vi "Draw Compass.vi"(5 "FcdVI Refnum":refnum<vi>, 7 "2D Picture":refnum<vi>, 9 "State in":T1={"Draw Options"={"Outer Border Color"=0, "Inner Border Color"=6316128, "Outer Gradient Color"=2565927, "Inner Gradient Color"=16860, "Compass North Pointer Color"=16711680, "Compass Pointer Color 1"=13355429, "Compass Pointer Color 2"=14934973, "Direction Pointer Color"=16765184, "Text Box Outline Color"=13355429, "Text Box Background Color"=14934973, "Scale Color"=16448250, "Text Color"=0, "Draw Gradient"=TRUE, "Draw Rose"=TRUE, "Simple Scale"=TRUE, "Draw Text"=FALSE, "Font Name"="Helvetica", "Angle Units"=enum."Degrees"}}, 10 "Data in":T4) -> (3 "picture out":picture)   [LabVIEW 2017, in "Compass Indicator.xctl"]
uses:
  <vilib>/robotics/Controls/Compass Indicator/Compass Indicator.xctl
  <vilib>/robotics/Controls/Compass Indicator/_Compass Indicator Support Files/Compass Data.ctl
  <vilib>/robotics/Controls/Compass Indicator/_Compass Indicator Support Files/Compass State.ctl
  <vilib>/robotics/Controls/Compass Indicator/Compass Picture/Draw Options.ctl
  <vilib>/robotics/Controls/Utilities/Angle Units.ctl
  <vilib>/Utility/miscctls.llb/LVBoundsTypeDef.ctl
  <vilib>/Utility/miscctls.llb/LVPositionTypeDef.ctl
  <vilib>/robotics/Controls/Compass Indicator/Compass Picture/NI_Robotics_Compass Picture.lvlib
  <vilib>/robotics/Controls/Utilities/NI_Robotics_Control Utilities.lvlib
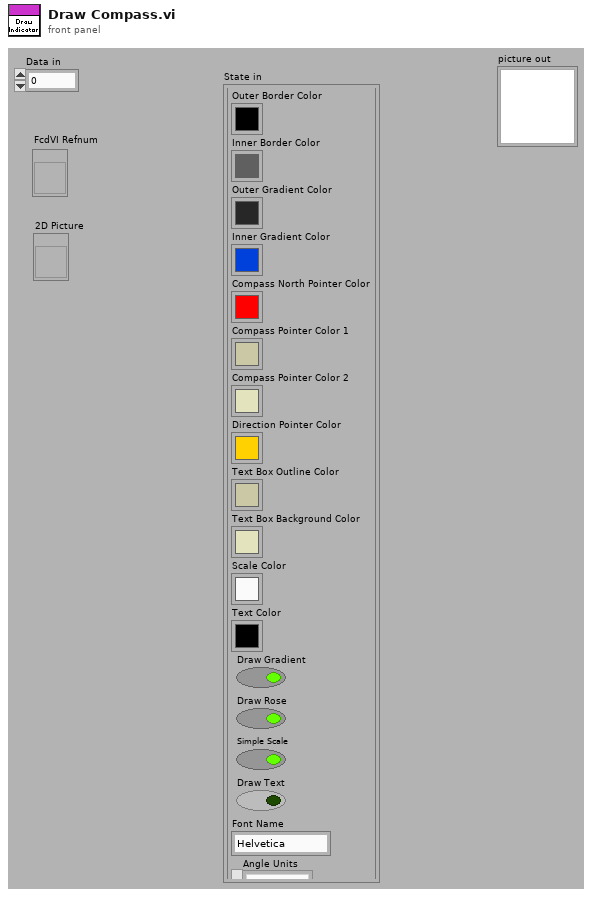
[diagram p1: front panel]
types:
  T1 = typedef "Compass Indicator.xctl/Compass State.ctl" = cluster{"Draw Options":T2}
  T2 = typedef "NI_Robotics_Compass Picture.lvlib/Draw Options.ctl" = cluster{"Outer Border Color":u32, "Inner Border Color":u32, "Outer Gradient Color":u32, "Inner Gradient Color":u32, "Compass North Pointer Color":u32, "Compass Pointer Color 1":u32, "Compass Pointer Color 2":u32, "Direction Pointer Color":u32, "Text Box Outline Color":u32, "Text Box Background Color":u32, "Scale Color":u32, "Text Color":u32, "Draw Gradient":bool, "Draw Rose":bool, "Simple Scale":bool, "Draw Text":bool, "Font Name":string, "Angle Units":T3}
  T3 = typedef "NI_Robotics_Control Utilities.lvlib/Angle Units.ctl" = enum16{"Radians", "Degrees"}
  T4 = typedef "Compass Indicator.xctl/Compass Data.ctl" = dbl
  T5 = typedef "LVPositionTypeDef.ctl" = cluster{"Left":i32, "Top":i32}
  T6 = typedef "LVBoundsTypeDef.ctl" = cluster{"Width":u32, "Height":u32}
  T7 = typedef "LVRectTypeDef.ctl" = cluster{"Left":i16, "Top":i16, "Right":i16, "Bottom":i16}
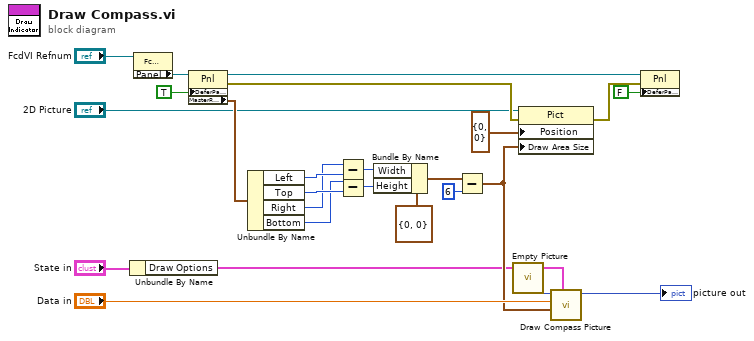
[diagram p0: block diagram]
diagram:
  n1 = Unbundle By Name("State in") -> ("Draw Options"=w1:T2)
  n2 = property class="FcdVI"(reference="FcdVI Refnum") -> ("Panel"=w10:refnum<vi>)  [unwired: 1 in, 2 out]
  n3 = property class="Pnl"(reference=w10, "DeferPanUpdts"=TRUE ("Defer Panel Updates")) -> (reference out=w12:refnum<vi>, error out=w14:errorcluster, "MasterRect"=w15:T7)  [unwired: 1 in]
  n4 = Unbundle By Name(w15) -> ("Left"=w17:i16, "Top"=w19:i16, "Right"=w16:i16, "Bottom"=w18:i16)
  n5 = Subtract(x=w16, y=w17) -> (x-y=w21:i16)
  n6 = Subtract(x=w18, y=w19) -> (x-y=w22:i16)
  n7 = Bundle By Name(cluster=T6 {"Width"=0, "Height"=0} ("Draw Area Size"), "Width"=w21, "Height"=w22) -> (w23:T6)
  n8 = Subtract(x=w23, y=u32 6) -> (x-y=w4:T6)
  n9 = call "Empty Picture"() -> ("empty picture"=w3:picture)
  n10 = property class="Pict"(reference="2D Picture", error in=w14, "Position"=T5 {"Left"=0, "Top"=0}, "Draw Area Size"=w4) -> (error out=w7:errorcluster)  [unwired: 1 out]
  n11 = call <vilib>:"Draw Compass Picture.vi"("draw options"=w1, "DrawAreaSize"=w4, "angle"="Data in", "picture in"=w3) -> ("picture out"=→"picture out":picture)  [unwired: 6 in, 1 out]
  n12 = property class="Pnl"(reference=w12, error in=w7, "DeferPanUpdts"=FALSE ("Defer Panel Updates")) -> ()  [unwired: 2 out]
